vi "Create All Message Queues.vi"(8 "error in (no error)":errorcluster) -> (0 "error out":errorcluster, 3 "Message Queues out":T1)   [LabVIEW 2017, in "Message Queue.lvlib"]
doc: "This VI creates and initializes all the message queues for your application. If your application requires more than one message queue, right-click the \"Message Queues\" constant above and select Open Type Def. Add the new Message Queue(s) to the type definition, then initialize them in this VI."
uses:
  Message Queue.lvlib
  All Message Queues.ctl
  Message Cluster.ctl
  Enqueue Message (Single).vi
  Global/Global refs.vi
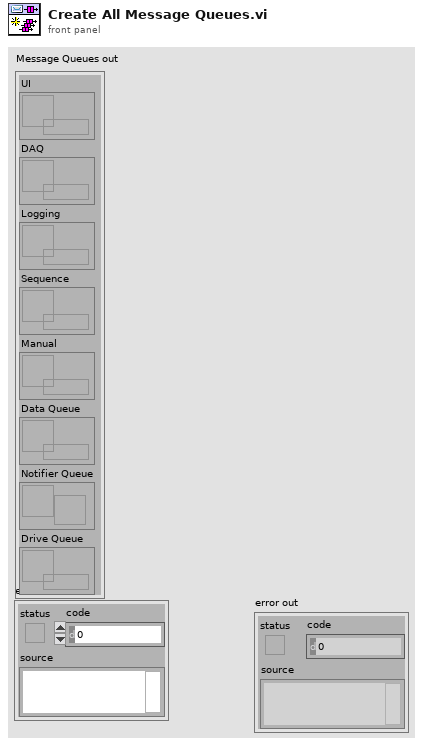
[diagram p1: front panel]
types:
  T1 = typedef "Message Queue.lvlib/All Message Queues.ctl" = cluster{"UI":refnum<queue>, "DAQ":refnum<queue>, "Logging":refnum<queue>, "Sequence":refnum<queue>, "Manual":refnum<queue>, "Data Queue":refnum<queue>, "Notifier Queue":refnum<notifier>, "Drive Queue":refnum<queue>}
  T2 = cluster{"UI":refnum<queue>, "DAQ":refnum<queue>, "Logging":refnum<queue>, "Sequence":refnum<queue>, "Manual":refnum<queue>}
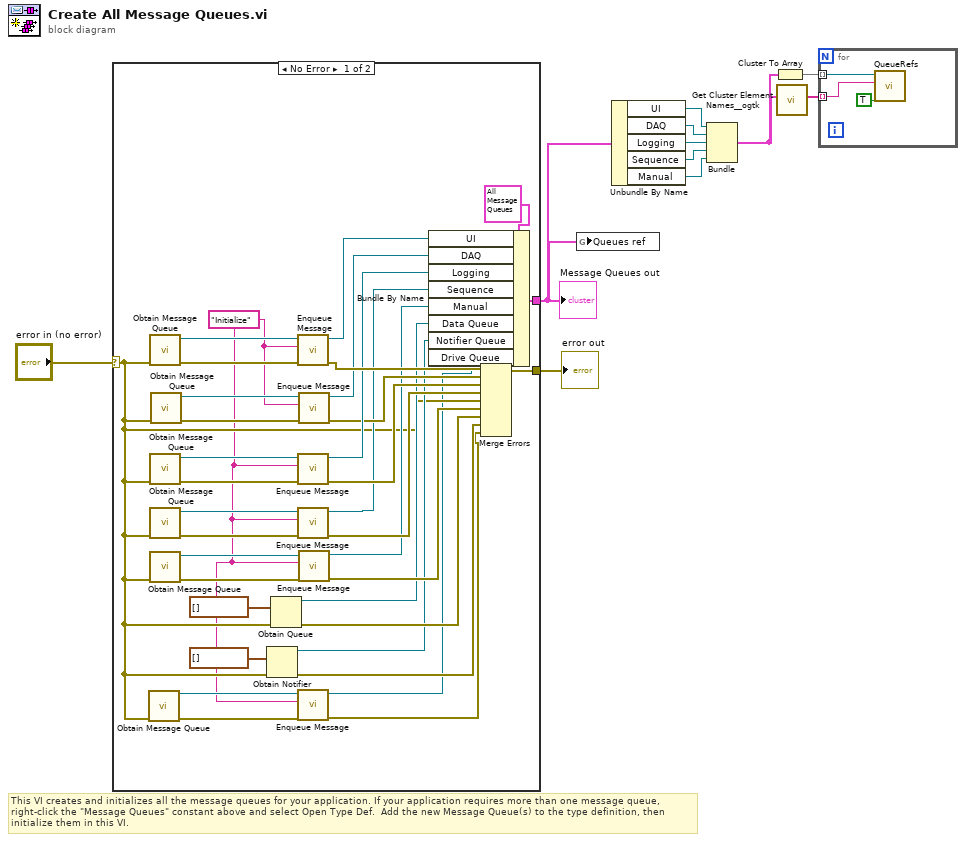
[diagram p0: block diagram]
diagram:
  # "This VI creates and initializes all the message queues for your application. If your application requires more than one message queue, right-click the \"Message Queues\" constant above and select Open Type Def.  Add the new Message Queue(s) to the type definition, then initialize them in this VI."
  n1 = case shown="No Error" "error in (no error)" {
    selector: "error in (no error)" -> [w16 w47]
    tunnel: [w34 w47] -> w11
    tunnel: [w44 _] -> w9
    frame No Error {
      w12 = "Initialize" ("Message")
      n2 = call "Obtain Message Queue.vi"("error in (no error)"=w16) -> ("error out"=w17:errorcluster, "Message Queue"=w14:refnum<queue>)  [unwired: 9 in]
      n3 = call "Obtain Message Queue.vi"("error in (no error)"=w16) -> ("error out"=w43:errorcluster, "Message Queue"=w42:refnum<queue>)  [unwired: 9 in]
      n4 = call "Obtain Message Queue.vi"("error in (no error)"=w16) -> ("error out"=w39:errorcluster, "Message Queue"=w38:refnum<queue>)  [unwired: 9 in]
      n5 = call "Obtain Message Queue.vi"("error in (no error)"=w16) -> ("error out"=w30:errorcluster, "Message Queue"=w31:refnum<queue>)  [unwired: 9 in]
      n6 = call "Obtain Message Queue.vi"("error in (no error)"=w16) -> ("error out"=w27:errorcluster, "Message Queue"=w25:refnum<queue>)  [unwired: 9 in]
      n7 = call "Obtain Message Queue.vi"("error in (no error)"=w16) -> ("error out"=w40:errorcluster, "Message Queue"=w41:refnum<queue>)  [unwired: 9 in]
      n8 = Obtain Notifier(notification data type=waveform(dbl)[] [], error in (no error)=w16) -> (notifier out=w20:refnum<notifier>, error out=w22:errorcluster)  [unwired: 2 in, 1 out]
      n9 = Obtain Queue(element data type=waveform(dbl)[] [], error in (no error)=w16) -> (queue out=w21:refnum<queue>, error out=w23:errorcluster)  [unwired: 3 in, 1 out]
      n10 = call-poly "Enqueue Message.vi"("error in (no error)"=w43, "Message"=w12, "Message Queue"=w42) -> ("error out"=w46:errorcluster, "dup Message Queue"=w37:refnum<queue>)  [unwired: 7 in]
      n11 = call-poly "Enqueue Message.vi"("error in (no error)"=w39, "Message"=w12, "Message Queue"=w38) -> ("error out"=w32:errorcluster, "dup Message Queue"=w35:refnum<queue>)  [unwired: 7 in]
      n12 = call-poly "Enqueue Message.vi"("error in (no error)"=w30, "Message"=w12, "Message Queue"=w31) -> ("error out"=w28:errorcluster, "dup Message Queue"=w29:refnum<queue>)  [unwired: 7 in]
      n13 = call-poly "Enqueue Message.vi"("error in (no error)"=w17, "Message"=w12, "Message Queue"=w14) -> ("error out"=w15:errorcluster, "dup Message Queue"=w13:refnum<queue>)  [unwired: 7 in]
      n14 = call-poly "Enqueue Message.vi"("error in (no error)"=w40, "Message"=w12, "Message Queue"=w41) -> ("error out"=w33:errorcluster, "dup Message Queue"=w36:refnum<queue>)  [unwired: 7 in]
      n15 = call-poly "Enqueue Message.vi"("error in (no error)"=w27, "Message"=w12, "Message Queue"=w25) -> ("error out"=w26:errorcluster, "dup Message Queue"=w24:refnum<queue>)  [unwired: 7 in]
      n16 = Bundle By Name(cluster=T1 {"UI"=refnum, "DAQ"=refnum, "Logging"=refnum, "Sequence"=refnum, "Manual"=refnum, "Data Queue"=refnum, "Notifier Queue"=refnum, "Drive Queue"=refnum} ("Message Queues"), "UI"=w37, "DAQ"=w36, "Logging"=w35, "Sequence"=w29, "Manual"=w24, "Data Queue"=w21, "Notifier Queue"=w20, "Drive Queue"=w13) -> (w44:T1)
      n17 = Merge Errors(w46, w33, w32, w28, w16, w26, w23, w22, w15) -> (w34:errorcluster)
    }
    frame Error {
    }
  }
  "Message Queues out" <- w9
  "error out" <- w11
  n18 = global write "Global refs.vi" "Queues ref"(w9) -> ()
  n19 = Unbundle By Name(w9) -> ("UI"=w8:refnum<queue>, "DAQ"=w7:refnum<queue>, "Logging"=w6:refnum<queue>, "Sequence"=w5:refnum<queue>, "Manual"=w4:refnum<queue>)
  n20 = Bundle("UI"=w8, "DAQ"=w7, "Logging"=w6, "Sequence"=w5, "Manual"=w4) -> (w3:T2)  [unwired: 1 in]
  n21 = Cluster To Array(cluster=w3) -> (array=w1:refnum<queue>[])
  n22 = call <userlib>:"Get Cluster Element Names__ogtk.vi"("Cluster"=w3) -> ("Element Names"=w2:string[])  [unwired: 9 in, 1 out]
  n23 = for {
    tunnel: w2 -> [w48] mode=indexing
    tunnel: w1 -> [w49] mode=indexing
    n24 = call "QueueRefs.vi"("Set?"=TRUE, "Queue Name"=w48, "Queue Ref"=w49) -> ()  [unwired: 8 in, 1 out]
  }
